vi "Destroy Session.vi"(8 "error in (no error)":errorcluster, 11 "advanced-http-client in":refnum<class "advanced-http-client.lvclass">) -> (0 "error out":errorcluster)   [LabVIEW 2020, in "advanced-http-client.lvclass"]
uses:
  advanced-http-client.lvclass
  advanced-http-client.lvclass/advanced-http-client.ctl
  <vilib>/NI/Advanced HTTP Client/Session.lvclass
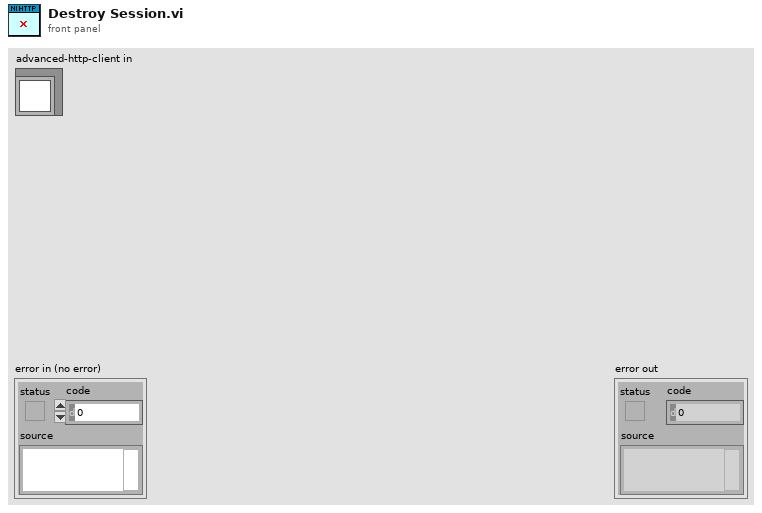
[diagram p1: front panel]
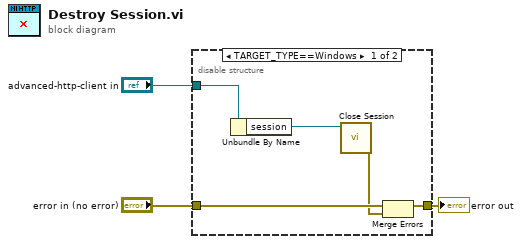
[diagram p0: block diagram]
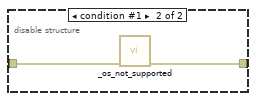
[diagram p2: hidden frame]
diagram:
  n1 = disable-structure shown="TARGET_TYPE==Windows" {
    disable-tunnel: "advanced-http-client in" -> [w4 _]
    disable-tunnel: [w8 w9] -> w2
    disable-tunnel: "error in (no error)" -> [w7 w10]
    frame condition #0 (active) {
      n2 = Unbundle By Name(w4) -> ("session"=w6:refnum<class "Session.lvclass">)
      n3 = call <vilib>:"Close Session.vi"("session"=w6) -> ("error out"=w5:errorcluster)  [unwired: 10 in]
      n4 = Merge Errors(w7, w5) -> (w8:errorcluster)
    }
    frame condition #1 {
      n5 = call "_os_not_supported.vi"("error in (no error)"=w10) -> ("error out"=w9:errorcluster)  [unwired: 9 in, 1 out]
    }
  }
  "error out" <- w2
